vi "SMTP Email Register Recipients.vi"(4 "error in (no error)":errorcluster, 6 "recipients":string[](array[string]), 7 "smtp session":T1) -> (0 "error out":errorcluster, 2 "invalid recipients":string[](array[string]), 3 "smtp session out":T1)   [LabVIEW 2011, in "NewNI_SMTPEmail.lvlib"]
doc: "This VI registers recipients of the mail with the SMTP server.\n\nSMTP Session: Descriptor of TCP connection the SMTP server.\n\nRecipients: An array of strings representing e-mail addresses of maiboxes of the recipients of the e-mail. Note that if one (or more) recipients fail to be recognized, the VI will keep registering the rest of the recipients until the array is exausted.\n\nInvalid Recipients: An array of recipients that were not recognized.\n\nerror out: error out cluster may contain an error string even though the status field is false. This happens in case of the error code 550 (unrecognized recipient) received from the SMTP server."
uses:
  NewNI_SMTPEmail.lvlib
  SMTP Email Session.ctl
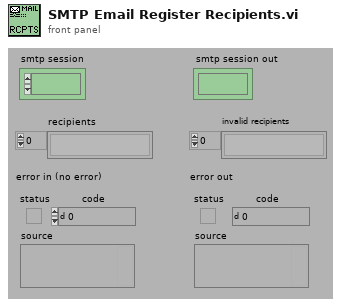
[diagram p1: front panel]
types:
  T1 = typedef "NewNI_SMTPEmail.lvlib/SMTP Email Session.ctl" = refnum<k1>
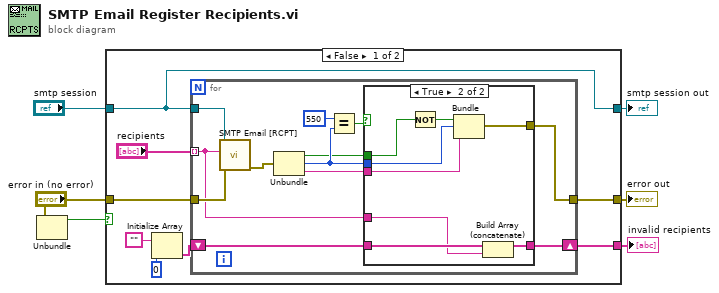
[diagram p0: block diagram]
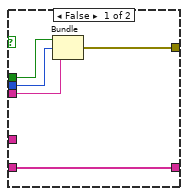
[diagram p2: hidden frame]
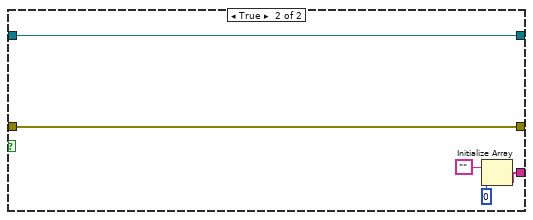
[diagram p3: hidden frame]
diagram:
  n1 = Unbundle("error in (no error)") -> ("status"=w5:bool)  [unwired: 2 out]
  n2 = case shown="False" w5 {
    tunnel: "error in (no error)" -> [w14 w44]
    tunnel: [w13 w44] -> w4
    tunnel: "smtp session" -> [w7 w43]
    tunnel: [w7 w43] -> w3
    tunnel: [w11 w40] -> w1
    frame False {
      n3 = Initialize Array("", 0) -> (w10:string[])
      n4 = for {
        tunnel: w14 -> [w26]
        tunnel: [w23] -> w13
        tunnel: w7 -> [w18]
        tunnel: "recipients" -> [w15] mode=indexing
        shift-right: [w16] -> w11
        shift-left: w10 -> [w17]
        n5 = call "SMTP Email [RCPT].vi"("error in (no error)"=w26, "address"=w15, "smtp session"=w18) -> ("error out"=w19:errorcluster)  [unwired: 1 in, 3 out]
        n6 = Unbundle(w19) -> ("status"=w20:bool, "code"=w21:i32, "source"=w22:string)
        n7 = Equal?(x=550, y=w21) -> (x = y?=w24:bool)
        n8 = case shown="True" w24 {
          tunnel: [w29 w39] -> w23
          tunnel: w22 -> [w30 w35]
          tunnel: w21 -> [w31 w38]
          tunnel: w20 -> [w28 w36]
          tunnel: w17 -> [w27 w34]
          tunnel: w15 -> [_ w33]
          tunnel: [w27 w32] -> w16
          frame False {
            n9 = Bundle("status"=w28, "code"=w31, "source"=w30) -> (w29:errorcluster)  [unwired: 1 out]
          }
          frame True {
            n10 = Not(x=w36) -> (.not. x?=w37:bool)
            n11 = Bundle(w37, "code"=w38, "source"=w35) -> (w39:cluster{bool, "code":i32, "source":string})  [unwired: 1 out]
            n12 = Build Array (concatenate)(w34, w33) -> (w32:string[])
          }
        }
      }
    }
    frame True {
      n13 = Initialize Array("", 0) -> (w40:string[])
    }
  }
  "smtp session out" <- w3
  "error out" <- w4
  "invalid recipients" <- w1
